vi "STS_Cal_RefData_Rescaling.vi"(8 "错误输入（无错误）":errorcluster, 11 "PDLSTS":refnum<k24>) -> (0 "error out":errorcluster, 3 "PDLSTS out":refnum<k24>)   [LabVIEW 2017]
doc: "Reference data rescaling"
uses:
  D:/test/PDLSTS/LV_PDL_Sample/DLL/STSProcess.dll
  DLL/STSProcess.dll
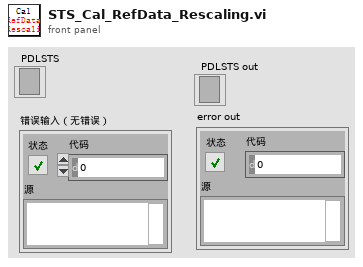
[diagram p1: front panel]
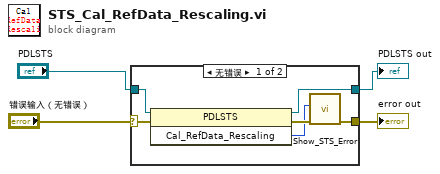
[diagram p0: block diagram]
diagram:
  n1 = case shown="无错误" "错误输入（无错误）" {
    selector: "错误输入（无错误）" -> [w9 w12]
    tunnel: "PDLSTS" -> [w10 w11]
    tunnel: [w6 w12] -> w2
    tunnel: [w5 w11] -> w1
    frame No Error {
      n2 = invoke class="PDLSTS" method="Cal_RefData_Rescaling"(reference=w10, error in=w9) -> (reference out=w5:refnum<k24>, error out=w8:errorcluster, "Cal_RefData_Rescaling"=w7:i32)  [unwired: 1 in]
      n3 = call "Show_STS_Error.vi"("error in (no error)"=w8, "Error"=w7) -> ("error out"=w6:errorcluster)  [unwired: 9 in]
    }
    frame Error {
    }
  }
  "error out" <- w2
  "PDLSTS out" <- w1
